vi "Create.vi"(7 "_Rescript in":refnum<class "_Rescript.lvclass">, 8 "error in":errorcluster) -> (0 "error out":errorcluster, 5 "_Rescript out":refnum<class "_Rescript.lvclass">)   [LabVIEW 2025, in "_Rescript.lvlib" / "Actor.lvlib"]
uses:
  Actor.lvlib
  _Rescript/_Rescript.lvclass
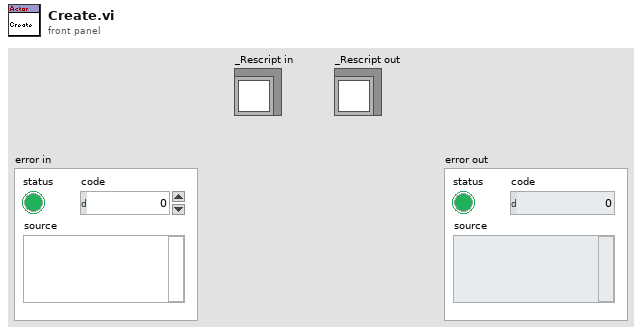
[diagram p1: front panel]
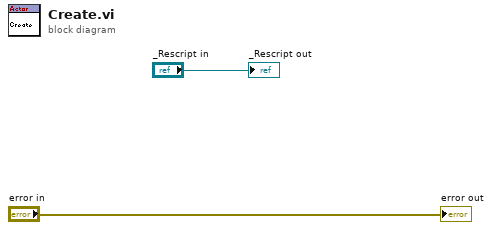
[diagram p0: block diagram]
diagram:
  "_Rescript out" <- "_Rescript in"
  "error out" <- "error in"
